vi "10_5.vi"() -> ()   [LabVIEW 2012]
panel:
  out "ADC Deviation":cluster{"Y":dbl[], "Y":dbl[]}[](graph)
  out "ADC Output":cluster{"Y":dbl[], "Y":dbl[]}[](graph)
  out "ADC Output":dbl
  out "ADC Input":dbl
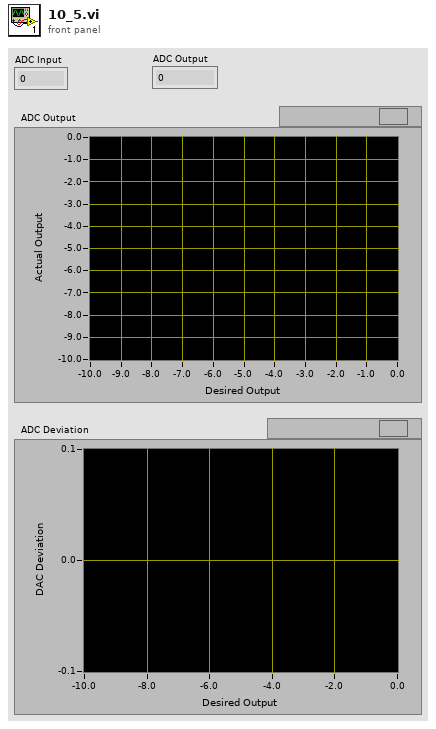
[diagram p1: front panel]
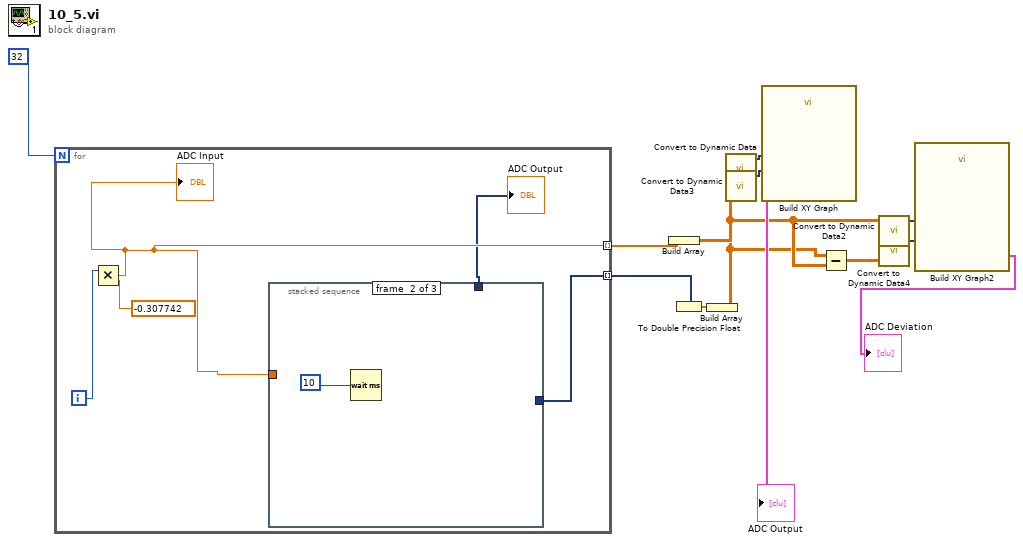
[diagram p0: block diagram]
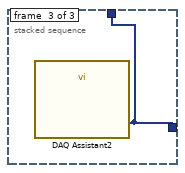
[diagram p3: hidden frame]
diagram:
  n1 = for {
    N: 32 -> [_]
    tunnel: [w16] -> w10 mode=indexing
    tunnel: [w15] -> w9 mode=indexing
    i -> [w17]
    n2 = Multiply(x=w17, y=-0.307742) -> (x*y=w16:dbl)
    "ADC Input" <- w16
    n3 = stacked-sequence {
      tunnel: w16 -> [_ _ _]
      tunnel: [_ _ w20] -> w14
      tunnel: [_ _ w20] -> w15
      frame #0 {
      }
      frame #1 {
        n4 = Wait (ms)(milliseconds to wait=u32 10) -> ()  [unwired: 1 out]
      }
      frame #2 {
        n5 = call "DAQ Assistant2"() -> ("data"=w20:dynamicdata)  [unwired: 17 in, 2 out]
      }
    }
    "ADC Output" <- w14
  }
  n6 = Build Array(w10) -> (w4:dbl[][])
  n7 = To Double Precision Float(number=w9) -> (double precision float=w7:dbl[])
  n8 = Build Array(w7) -> (w3:dbl[][])
  n9 = call "Convert to Dynamic Data"("2D Array"=w4) -> ("Dynamic Data Type"=w6:dynamicdata)  [unwired: 3 in]
  n10 = call "Convert to Dynamic Data3"("2D Array"=w3) -> ("Dynamic Data Type"=w8:dynamicdata)  [unwired: 3 in]
  n11 = call "Build XY Graph"("Y Input"=w8, "X Input"=w6) -> ("XY Graph"=→"ADC Output":cluster{"Y":dbl[], "Y":dbl[]}[])  [unwired: 3 in, 6 out]
  n12 = Subtract(x=w3, y=w4) -> (x-y=w2:dbl[][])
  n13 = call "Convert to Dynamic Data2"("2D Array"=w4) -> ("Dynamic Data Type"=w5:dynamicdata)  [unwired: 3 in]
  n14 = call "Convert to Dynamic Data4"("2D Array"=w2) -> ("Dynamic Data Type"=w1:dynamicdata)  [unwired: 3 in]
  n15 = call "Build XY Graph2"("Y Input"=w1, "X Input"=w5) -> ("XY Graph"=→"ADC Deviation":cluster{"Y":dbl[], "Y":dbl[]}[])  [unwired: 3 in, 6 out]
